vi "Write Image Header.vi"(8 "error in (no error)":errorcluster, 11 "Save Image in":refnum<class "Save Image.lvclass">) -> (0 "error out":errorcluster, 3 "Save Image out":refnum<class "Save Image.lvclass">)   [LabVIEW 2018, in "Save Image.lvclass"]
uses:
  Save Image.lvclass
  Save Image.lvclass/Save Image.ctl
  Header/Header.lvclass/Header.ctl
  <userlib>/gfitsio/gfitsio-write-key-string.vi
  <userlib>/gfitsio/gfitsio.lvlib
  Header/Header.lvclass
panel:
  out "SERN":T1
  out "Header Contents":T2
types:
  T1 = cluster{"Name":string, "Value":string, "Comment":string}
  T2 = cluster{"FILENAME":cluster{"Name":string, "Value":string, "Comment":string}, "OBSERVER":cluster{"Name":string, "Value":string, "Comment":string}, "PROGRID":cluster{"Name":string, "Value":string, "Comment":string}, "OBJECT":cluster{"Name":string, "Value":string, "Comment":string}, "NIGHTDIR":cluster{"Name":string, "Value":string, "Comment":string}, "CHANNEL":cluster{"Name":string, "Value":string, "Comment":string}, "INSTRUME":cluster{"Name":string, "Value":string, "Comment":string}, "NEXPSEQ":cluster{"Name":string, "Value":string, "Comment":string}, "SEQINDEX":cluster{"Name":string, "Value":string, "Comment":string}, "OBSTYPE":cluster{"Name":string, "Value":string, "Comment":string}, "READMOD":cluster{"Name":string, "Value":string, "Comment":string}, "READMODE":cluster{"Name":string, "Value":string, "Comment":string}, "ACQMODE":cluster{"Name":string, "Value":string, "Comment":string}, "PREAMP":cluster{"Name":string, "Value":string, "Comment":string}, "READOUT":cluster{"Name":string, "Value":string, "Comment":string}, "VSHIFT":cluster{"Name":string, "Value":string, "Comment":string}, "TRIGGER":cluster{"Name":string, "Value":string, "Comment":string}, "EMMODE":cluster{"Name":string, "Value":string, "Comment":string}, "EMGAIN":cluster{"Name":string, "Value":string, "Comment":string}, "VBIN":cluster{"Name":string, "Value":string, "Comment":string}, "HBIN":cluster{"Name":string, "Value":string, "Comment":string}, "INITLIN":cluster{"Name":string, "Value":string, "Comment":string}, "INITCOL":cluster{"Name":string, "Value":string, "Comment":string}, "FINALLIN":cluster{"Name":string, "Value":string, "Comment":string}, "FINALCOL":cluster{"Name":string, "Value":string, "Comment":string}, "KSERLEN":cluster{"Name":string, "Value":string, "Comment":string}, "SHUTTER":cluster{"Name":string, "Value":string, "Comment":string}, "OPENSHT":cluster{"Name":string, "Value":string, "Comment":string}, "CLOSESHT":cluster{"Name":string, "Value":string, "Comment":string}, "DATE":cluster{"Name":string, "Value":string, "Comment":string}, "GAIN":cluster{"Name":string, "Value":string, "Comment":string}, "GAINERR":cluster{"Name":string, "Value":string, "Comment":string}, "RDNOISE":cluster{"Name":string, "Value":string, "Comment":string}, "RNOISERR":cluster{"Name":string, "Value":string, "Comment":string}, "SKYFIBER":cluster{"Name":string, "Value":string, "Comment":string}, "CALFIBER":cluster{"Name":string, "Value":string, "Comment":string}, "UTDATE":cluster{"Name":string, "Value":string, "Comment":string}, "LOCTIME":cluster{"Name":string, "Value":string, "Comment":string}, "MJD":cluster{"Name":string, "Value":string, "Comment":string}, "OBSLON":cluster{"Name":string, "Value":string, "Comment":string}, "OBSLAT":cluster{"Name":string, "Value":string, "Comment":string}, "OBSALT":cluster{"Name":string, "Value":string, "Comment":string}, "EXPTIME":cluster{"Name":string, "Value":string, "Comment":string}, "TELRA":cluster{"Name":string, "Value":string, "Comment":string}, "TELDEC":cluster{"Name":string, "Value":string, "Comment":string}, "RA":cluster{"Name":string, "Value":string, "Comment":string}, "DEC":cluster{"Name":string, "Value":string, "Comment":string}, "RA_DEG":cluster{"Name":string, "Value":string, "Comment":string}, "DEC_DEG":cluster{"Name":string, "Value":string, "Comment":string}, "EPOCH":cluster{"Name":string, "Value":string, "Comment":string}, "HA":cluster{"Name":string, "Value":string, "Comment":string}, "HAD":cluster{"Name":string, "Value":string, "Comment":string}, "AIRMASS":cluster{"Name":string, "Value":string, "Comment":string}, "AMSTART":cluster{"Name":string, "Value":string, "Comment":string}, "AMEND":cluster{"Name":string, "Value":string, "Comment":string}, "XOFFSET":cluster{"Name":string, "Value":string, "Comment":string}, "YOFFSET":cluster{"Name":string, "Value":string, "Comment":string}, "PA":cluster{"Name":string, "Value":string, "Comment":string}, "CAMFOC":cluster{"Name":string, "Value":string, "Comment":string}, "TELFOC":cluster{"Name":string, "Value":string, "Comment":string}, "TCSUT":cluster{"Name":string, "Value":string, "Comment":string}, "TCSST":cluster{"Name":string, "Value":string, "Comment":string}, "MOONDIST":cluster{"Name":string, "Value":string, "Comment":string}, "MOONALT":cluster{"Name":string, "Value":string, "Comment":string}, "MOONPHAS":cluster{"Name":string, "Value":string, "Comment":string}, "ADC":cluster{"Name":string, "Value":string, "Comment":string}, "ADCSPEED":cluster{"Name":string, "Value":string, "Comment":string}, "CALMIRR":cluster{"Name":string, "Value":string, "Comment":string}, "GUIDING":cluster{"Name":string, "Value":string, "Comment":string}, "GUIDTEXP":cluster{"Name":string, "Value":string, "Comment":string}, "GUIDFREQ":cluster{"Name":string, "Value":string, "Comment":string}, "GUIDOBJX":cluster{"Name":string, "Value":string, "Comment":string}, "GUIDOBJY":cluster{"Name":string, "Value":string, "Comment":string}, "AVGYCORR":cluster{"Name":string, "Value":string, "Comment":string}, "AVGXCORR":cluster{"Name":string, "Value":string, "Comment":string}, "GFOCUS":cluster{"Name":string, "Value":string, "Comment":string}, "THARLAMP":cluster{"Name":string, "Value":string, "Comment":string}, "HALLAMP":cluster{"Name":string, "Value":string, "Comment":string}, "AGITATOR":cluster{"Name":string, "Value":string, "Comment":string}, "THARMIRR":cluster{"Name":string, "Value":string, "Comment":string}, "DSTATUS":cluster{"Name":string, "Value":string, "Comment":string}, "DPOS":cluster{"Name":string, "Value":string, "Comment":string}, "DTEMP":cluster{"Name":string, "Value":string, "Comment":string}, "DHUM":cluster{"Name":string, "Value":string, "Comment":string}, "DLAMP":cluster{"Name":string, "Value":string, "Comment":string}, "DFLAT":cluster{"Name":string, "Value":string, "Comment":string}, "TEMPEXT":cluster{"Name":string, "Value":string, "Comment":string}, "PRESSURE":cluster{"Name":string, "Value":string, "Comment":string}, "HUMIDITY":cluster{"Name":string, "Value":string, "Comment":string}, "WINDDIR":cluster{"Name":string, "Value":string, "Comment":string}, "WINSPEED":cluster{"Name":string, "Value":string, "Comment":string}, "SHTTTL":cluster{"Name":string, "Value":string, "Comment":string}, "COOLER":cluster{"Name":string, "Value":string, "Comment":string}, "TEMP":cluster{"Name":string, "Value":string, "Comment":string}, "TEMPST":cluster{"Name":string, "Value":string, "Comment":string}, "SERN":cluster{"Name":string, "Value":string, "Comment":string}}
  T3 = enum16{"open", "open or create", "create or replace", "create", "open (read only)"}
  T4 = typedef "gfitsio.lvlib/gfitsio-refnum.ctl" = refnum<k1>
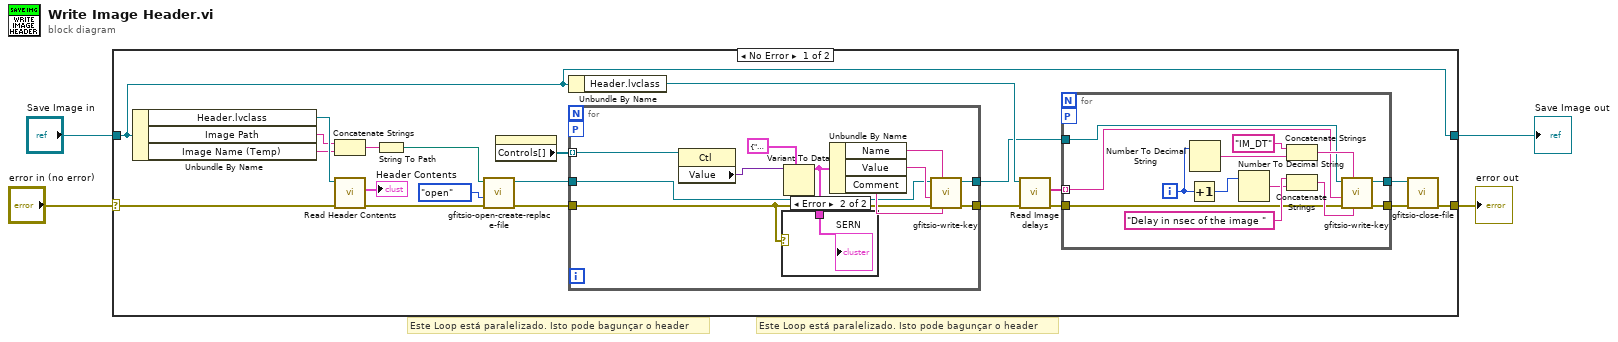
[diagram p0: block diagram]
diagram:
  # "Este Loop está paralelizado. Isto pode bagunçar o header"
  # "Este Loop está paralelizado. Isto pode bagunçar o header"
  n1 = case shown="No Error" "error in (no error)" {
    selector: "error in (no error)" -> [w21 w52]
    tunnel: [w17 w52] -> w3
    tunnel: [w15 w51] -> w1
    tunnel: "Save Image in" -> [w15 w51]
    frame No Error {
      n2 = Unbundle By Name(w15) -> ("Header.lvclass"=w22:refnum<class "Header.lvclass">, "Image Path"=w19:string, "Image Name (Temp)"=w18:string)
      n3 = Concatenate Strings(w19, w18) -> (w25:string)
      n4 = call "Read Header Contents.vi"("error in (no error)"=w21, "Header in"=w22) -> ("error out"=w20:errorcluster, "Header Content"=→"Header Contents":T2)  [unwired: 7 in, 1 out]
      n5 = String To Path(string=w25) -> (path=w24:path)
      n6 = call <userlib>:"gfitsio-open-create-replace-file.vi"("error in (no error)"=w20, "function (open)"=T3."open", "file path (dialog if empty)"=w24) -> ("error out"=w5:errorcluster, "gfits refnum"=w6:T4)  [unwired: 6 in, 1 out]
      n7 = property on="Header Contents" class="Clust (strict)"() -> ("Controls[]"=w9:refnum<vi>[])  [unwired: 2 in, 2 out]
      n8 = Unbundle By Name(w15) -> ("Header.lvclass"=w14:refnum<class "Header.lvclass">)
      n9 = for {
        tunnel: w9 -> [w47] mode=indexing
        tunnel: w6 -> [w42]
        tunnel: [w41] -> w8
        tunnel: w5 -> [w40]
        tunnel: [w49] -> w12
        workers-P: _ -> [_]
        n10 = property class="Ctl"(reference=w47) -> ("Value"=w48:variant)  [unwired: 1 in, 2 out]
        n11 = Variant To Data(type=T1 {"Name"="", "Value"="", "Comment"=""} ("SERN"), Variant=w48) -> (data=w39:T1)  [unwired: 1 in, 1 out]
        n12 = case shown="Error" w40 {
          tunnel: w39 -> [_ w50]
          frame No Error {
          }
          frame Error {
            "SERN" <- w50
          }
        }
        n13 = Unbundle By Name(w39) -> ("Name"=w45:string, "Value"=w44:string, "Comment"=w43:string)
        n14 = call-poly <userlib>:"gfitsio-write-key.vi"("comment"=w43, "keyname"=w45, "error in (no error)"=w40, "value"=w44, "gfits refnum"=w42) -> ("error out"=w49:errorcluster, "dup gfits refnum"=w41:T4)  [unwired: 5 in]
      }
      n15 = call "Read Image delays.vi"("error in (no error)"=w12, "Header in"=w14) -> ("error out"=w13:errorcluster, "Image delays"=w11:string[])  [unwired: 7 in, 1 out]
      n16 = for {
        tunnel: w11 -> [w35] mode=indexing
        tunnel: w8 -> [w28]
        tunnel: [w27] -> w7
        tunnel: w13 -> [w26]
        tunnel: [w31] -> w16
        workers-P: _ -> [_]
        i -> [w33]
        n17 = Increment(x=w33) -> (x+1=w34:i32)
        n18 = Number To Decimal String(number=w33) -> (decimal integer string=w37:string)  [unwired: 1 in]
        n19 = Number To Decimal String(number=w34) -> (decimal integer string=w29:string)  [unwired: 1 in]
        n20 = Concatenate Strings("IM_DT", w37) -> (w36:string)
        n21 = Concatenate Strings("Delay in nsec of the image " ("comment"), w29) -> (w32:string)
        n22 = call-poly <userlib>:"gfitsio-write-key.vi"("comment"=w32, "keyname"=w36, "error in (no error)"=w26, "value"=w35, "gfits refnum"=w28) -> ("error out"=w31:errorcluster, "dup gfits refnum"=w27:T4)  [unwired: 5 in]
      }
      n23 = call <userlib>:"gfitsio-close-file.vi"("error in (no error)"=w16, "gfits refnum"=w7) -> ("error out"=w17:errorcluster)  [unwired: 8 in, 1 out]
    }
    frame Error {
    }
  }
  "error out" <- w3
  "Save Image out" <- w1
